vi "Set IP DHCP.vi"(8 "error in":errorcluster, 11 "MAC Address":string) -> (0 "error out":errorcluster, 3 "Network Module Information":T1 {"IP Mode" items=["Static"=1, "DHCP/Link-Local"=2, "Link-Local Only"=4, "DHCP Only"=8]})   [LabVIEW 2013]
uses:
  types/MAX Sys Cfg Target Information.ctl
  <vilib>/nisyscfg/Initialize (String).vi
  <vilib>/nisyscfg/Save Changes (System).vi
  <vilib>/nisyscfg/Close (System).vi
  <resource>/objmgr/nisysapi.rc
  <vilib>/nisyscfg/nisyscfg.lvlib
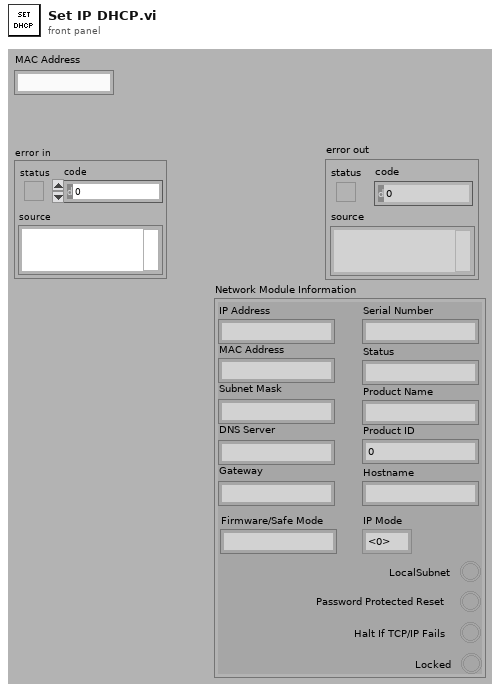
[diagram p1: front panel]
types:
  T1 = typedef "MAX Sys Cfg Target Information.ctl" = cluster{"MAC Address":string, "IP Address":string, "Status":string, "Product Name":string, "Hostname":string, "Firmware/Safe Mode":string, "Subnet Mask":string, "Gateway":string, "DNS Server":string, "Serial Number":string, "Product ID":u32, "Locked ":bool, "LocalSubnet":bool, "Halt If TCP/IP Fails":bool, "Password Protected Reset":bool, "IP Mode":i32}
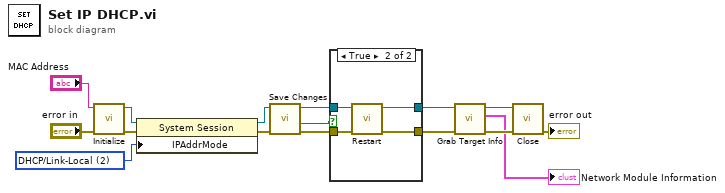
[diagram p0: block diagram]
diagram:
  w6 = 2 items=["Static"=1, "DHCP/Link-Local"=2, "Link-Local Only"=4, "DHCP Only"=8] ("Primary NIC:IP Address Request Mode")
  n1 = call-poly <vilib>:"Initialize.vi"("error in (no error)"="error in", "target (localhost)"="MAC Address") -> ("error out"=w12:errorcluster, "session out"=w11:refnum<k21>)  [unwired: 7 in, 1 out]
  n2 = property class="System Session"(reference=w11, error in=w12, "IPAddrMode"=w6) -> (reference out=w15:refnum<k21>, error out=w16:errorcluster)
  n3 = call-poly <vilib>:"Save Changes.vi"("error in (no error)"=w16, "session in"=w15) -> ("error out"=w14:errorcluster, "changes require restart"=w7:bool, "session out"=w13:refnum<k21>)  [unwired: 6 in, 1 out]
  n4 = case shown="True" w7 {
    tunnel: w14 -> [w18 w22]
    tunnel: w13 -> [w17 w21]
    tunnel: [w17 w20] -> w4
    tunnel: [w18 w19] -> w5
    frame False {
    }
    frame True {
      n5 = call <vilib>:"Restart.vi"("error in (no error)"=w22, "session in"=w21) -> ("error out"=w19:errorcluster, "session out"=w20:refnum<k21>)  [unwired: 7 in, 1 out]
    }
  }
  n6 = call "Grab Target Info.vi"("error in (no error)"=w5, "Refnum in"=w4) -> ("error out"=w2:errorcluster, "Network Module Information"=→"Network Module Information":T1, "Refnum out"=w3:refnum<k21>)  [unwired: 7 in]
  n7 = call-poly <vilib>:"Close.vi"("error in (no error)"=w2, "session in"=w3) -> ("error out"=→"error out":errorcluster)  [unwired: 9 in]
